vi "Disabled - Select Auto (SubVI).vi"(4 "lower limit":dbl=2.0 format="%#_13g", 6 "upper limit":dbl format="%#_13g", 10 "Increment":bool, 11 "Decrement":bool) -> (3 "Select Auto To Change":dbl)   [LabVIEW 2015]
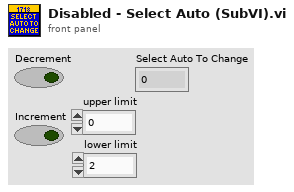
[diagram p1: front panel]
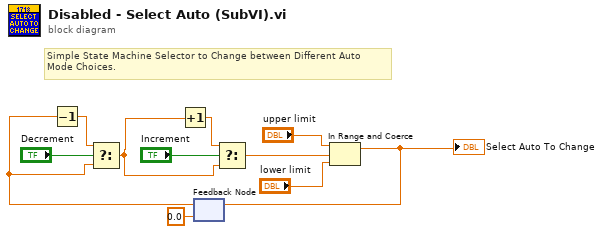
[diagram p0: block diagram]
diagram:
  # "Simple State Machine Selector to Change between Different Auto\nMode Choices."
  n1 = feedback #1(0.0) -> (w6:dbl)
  n2 = Decrement(x=w6) -> (x-1=w4:dbl)
  n3 = Select(t=w4, s="Decrement", f=w6) -> (s? t:f=w5:dbl)
  n4 = Increment(x=w5) -> (x+1=w3:dbl)
  n5 = Select(t=w3, s="Increment", f=w5) -> (s? t:f=w9:dbl)
  n6 = In Range and Coerce(upper limit="upper limit", x=w9, lower limit="lower limit") -> (coerced(x)=w1:dbl)  [unwired: 1 out]
  "Select Auto To Change" <- w1
  n7 = feedback-in #1(w1) -> ()
